vi "GetLimsTestStep.vi"(8 "error in (no error)":errorcluster, 10 "step-id":i32, 11 "ByteGSAPIBase in":refnum<class "ByteGSAPIBase.lvclass">) -> (0 "error out":errorcluster, 2 "StepList":T1, 3 "ByteGSAPIBase out":refnum<class "ByteGSAPIBase.lvclass">)   [LabVIEW 2019, in "ByteGSWebAPI.lvlib" / "ByteGSAPIBase.lvclass"]
doc: "Obtain a single step based on the step-id"
uses:
  ByteGSAPIBase.lvclass
  TypeDef/Step.ctl
  TypeDef/Asset.ctl
  ByteGSAPIBase.lvclass/ByteGSAPIBase.ctl
  <vilib>/Bytelabs/ByteREST/ByteRESTClass/ByteRESTBase/RESTBase.lvclass
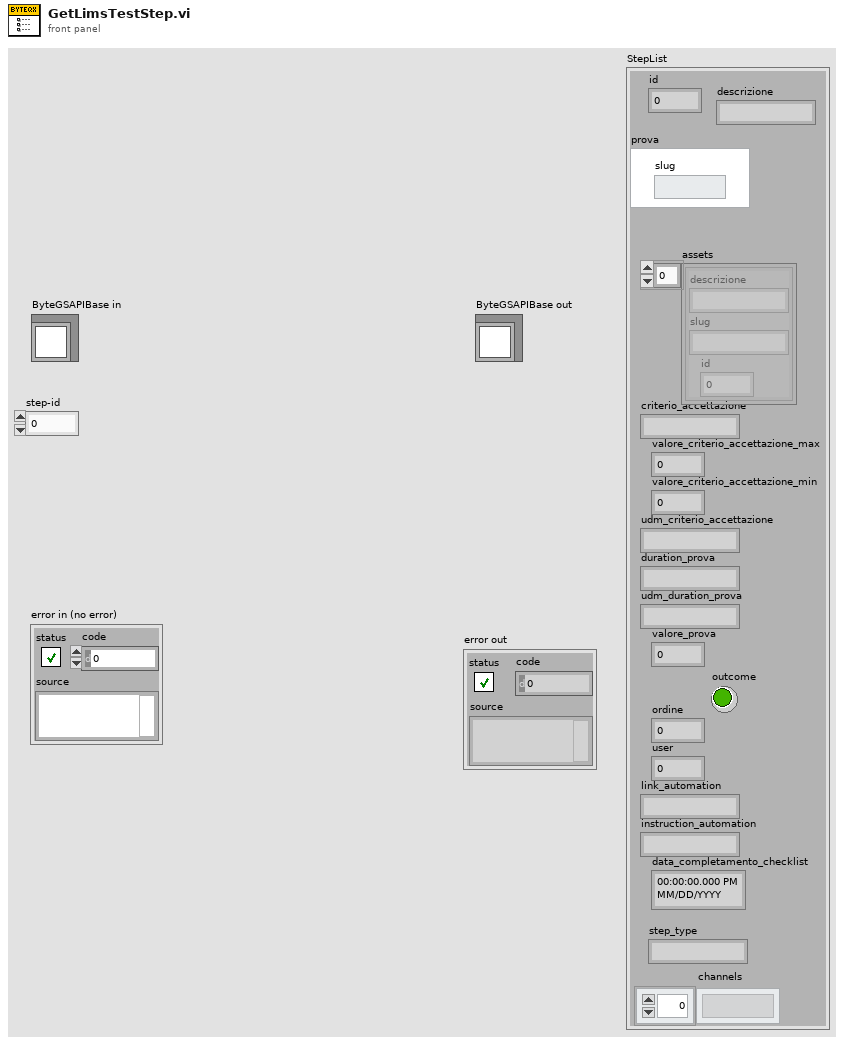
[diagram p1: front panel]
types:
  T1 = typedef "ByteGSWebAPI.lvlib/ByteGSAPIBase.lvclass/Step.ctl" = cluster{"id":i32, "descrizione":string, "prova":cluster{"slug":string}, "assets":T2[], "criterio_accettazione":string, "valore_criterio_accettazione_max":dbl, "valore_criterio_accettazione_min":dbl, "udm_criterio_accettazione":string, "duration_prova":string, "udm_duration_prova":string, "valore_prova":dbl, "ordine":i32, "user":i32, "link_automation":string, "instruction_automation":string, "data_completamento_checklist":timestamp, "outcome":bool, "step_type":string, "channels":string[]}
  T2 = typedef "ByteGSWebAPI.lvlib/ByteGSAPIBase.lvclass/Asset.ctl" = cluster{"descrizione":string, "slug":string, "id":i32}
  T3 = cluster{"id":i32, "descrizione":string, "assets":T2[], "criterio_accettazione":string, "valore_criterio_accettazione_max":dbl, "valore_criterio_accettazione_min":dbl, "udm_criterio_accettazione":string, "duration_prova":string, "udm_duration_prova":string, "data_completamento_checklist":string, "valore_prova":dbl, "outcome":string, "ordine":i32, "user":i32, "link_automation":string, "instruction_automation":string, "channels":string[], "step_type":string, "prova":cluster{"slug":string}}[]
  T4 = cluster{"id":i32, "descrizione":string, "assets":T2[], "criterio_accettazione":string, "valore_criterio_accettazione_max":dbl, "valore_criterio_accettazione_min":dbl, "udm_criterio_accettazione":string, "duration_prova":string, "udm_duration_prova":string, "data_completamento_checklist":string, "valore_prova":dbl, "outcome":string, "ordine":i32, "user":i32, "link_automation":string, "instruction_automation":string, "channels":string[], "step_type":string, "prova":cluster{"slug":string}}
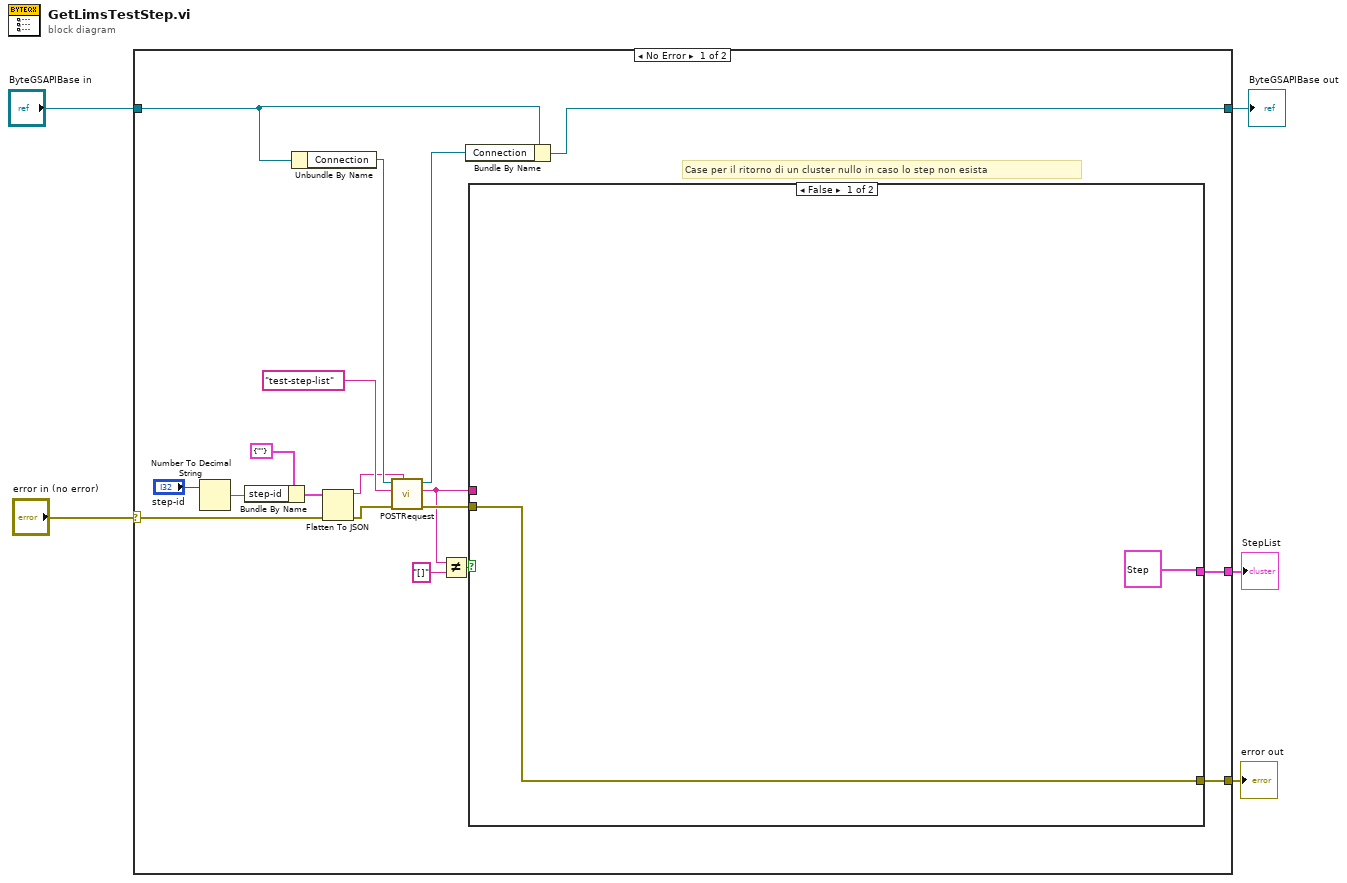
[diagram p0: block diagram]
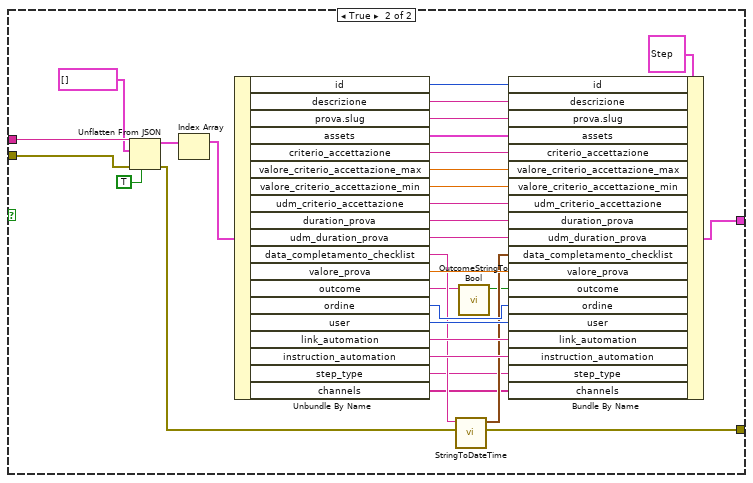
[diagram p2: hidden frame]
diagram:
  n1 = case shown="No Error" "error in (no error)" {
    selector: "error in (no error)" -> [w13 w58]
    tunnel: [w10 w58] -> w4
    tunnel: [w20 w57] -> w2
    tunnel: "ByteGSAPIBase in" -> [w21 w57]
    tunnel: [w9 _] -> w1
    frame No Error {
      # "Case per il ritorno di un cluster nullo in caso lo step non esista"
      n2 = Number To Decimal String(number="step-id") -> (decimal integer string=w17:string)  [unwired: 1 in]
      n3 = Bundle By Name(cluster=cluster{"step-id":string} {"step-id"=""} ("Request"), "step-id"=w17) -> (w15:cluster{"step-id":string})
      n4 = Unbundle By Name(w21) -> ("Connection"=w23:refnum<class "RESTBase.lvclass">)
      n5 = Flatten To JSON(anything=w15, error in (no error)=w13) -> (JSON string=w14:string, 11:w12:errorcluster)  [unwired: 1 in]
      n6 = call-dynamic "POSTRequest.vi"("Body in"=w14, "error in (no error)"=w12, "Request"="test-step-list", "ByteRESTBase in"=w23) -> ("error out"=w11:errorcluster, "Body"=w7:string, "ByteRESTBase out"=w22:refnum<class "RESTBase.lvclass">)  [unwired: 4 in, 1 out]
      n7 = Not Equal?(x=w7, y="[]") -> (x != y?=w8:bool)
      n8 = Bundle By Name(cluster=w21, "Connection"=w22) -> (w20:refnum<class "ByteGSAPIBase.lvclass">)
      n9 = case shown="False" w8 {
        tunnel: w7 -> [_ w56]
        tunnel: w11 -> [w25 w55]
        tunnel: [w25 w37] -> w10
        tunnel: [T1 {"id"=0, "descrizione"="", "prova"={"slug"=""}, "assets"=[], "criterio_accettazione"="", "valore_criterio_accettazione_max"=0.0, "valore_criterio_accettazione_min"=0.0, "udm_criterio_accettazione"="", "duration_prova"="", "udm_duration_prova"="", "valore_prova"=0.0, "ordine"=0, "user"=0, "link_automation"="", "instruction_automation"="", "data_completamento_checklist"=timestamp(0 s since 1904-01-01), "outcome"=FALSE, "step_type"="", "channels"=[]} ("StepList") w34] -> w9
        frame False {
        }
        frame True {
          n10 = Unflatten From JSON(JSON string=w56, type and defaults=T3 [], default null elements? (F)=TRUE, error in (no error)=w55) -> (value=w31:T3, error out=w36:errorcluster)  [unwired: 3 in]
          n11 = Index Array(array=w31) -> (element=w32:T4)  [unwired: 1 in]
          n12 = Unbundle By Name(w32) -> ("id"=w38:i32, "descrizione"=w39:string, "prova.slug"=w40:string, "assets"=w41:T2[], "criterio_accettazione"=w42:string, "valore_criterio_accettazione_max"=w43:dbl, "valore_criterio_accettazione_min"=w44:dbl, "udm_criterio_accettazione"=w45:string, "duration_prova"=w46:string, "udm_duration_prova"=w47:string, "data_completamento_checklist"=w48:string, "valore_prova"=w50:dbl, "outcome"=w29:string, "ordine"=w51:i32, "user"=w52:i32, "link_automation"=w53:string, "instruction_automation"=w54:string, "step_type"=w27:string, "channels"=w26:string[])
          n13 = call "StringToDateTime.vi"("error in (no error)"=w36, "datetime string"=w48) -> ("error out"=w37:errorcluster, "timestamp"=w49:timestamp)  [unwired: 8 in]
          n14 = call "OutcomeStringToBool.vi"("outcome string"=w29) -> ("outcome bool"=w28:bool)  [unwired: 10 in]
          n15 = Bundle By Name(cluster=T1 {"id"=0, "descrizione"="", "prova"={"slug"=""}, "assets"=[], "criterio_accettazione"="", "valore_criterio_accettazione_max"=0.0, "valore_criterio_accettazione_min"=0.0, "udm_criterio_accettazione"="", "duration_prova"="", "udm_duration_prova"="", "valore_prova"=0.0, "ordine"=0, "user"=0, "link_automation"="", "instruction_automation"="", "data_completamento_checklist"=timestamp(0 s since 1904-01-01), "outcome"=FALSE, "step_type"="", "channels"=[]} ("StepList"), "id"=w38, "descrizione"=w39, "prova.slug"=w40, "assets"=w41, "criterio_accettazione"=w42, "valore_criterio_accettazione_max"=w43, "valore_criterio_accettazione_min"=w44, "udm_criterio_accettazione"=w45, "duration_prova"=w46, "udm_duration_prova"=w47, "data_completamento_checklist"=w49, "valore_prova"=w50, "outcome"=w28, "ordine"=w51, "user"=w52, "link_automation"=w53, "instruction_automation"=w54, "step_type"=w27, "channels"=w26) -> (w34:T1)
        }
      }
    }
    frame Error {
    }
  }
  "error out" <- w4
  "ByteGSAPIBase out" <- w2
  "StepList" <- w1
